vi "行列加减.vi"(10 "减":i32, 11 "加":dbl) -> (0 "x-3":i32, 1 "x-4":i32, 2 "x+4":dbl, 3 "x+3":dbl, 4 "x-2":i32, 5 "x+2":dbl, 6 "x-1":i32, 7 "x+1":dbl)   [LabVIEW 2018]
doc: "将行或列的索引位置进行加减以达到索引当前点周围点的目的。\n比如当前行列分别为5、5，为了查询它上一行同一列的点即4行5列的棋子，将其行减一变为4，列保持不变即为5。其它点同理对其进行索引。\n因要多次引用这个VI，因此加减的功能合在一个VI里面以供调用。"
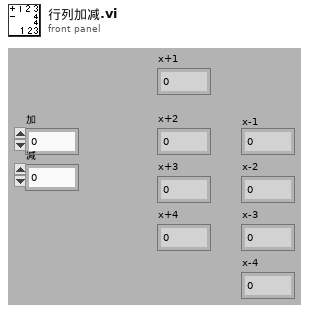
[diagram p1: front panel]
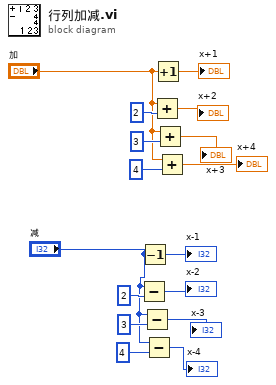
[diagram p0: block diagram]
diagram:
  n1 = Subtract(x="减", y=u8 2) -> (x-y=→"x-2":i32)
  n2 = Decrement(x="减") -> (x-1=→"x-1":i32)
  n3 = Subtract(x="减", y=u8 3) -> (x-y=→"x-3":i32)
  n4 = Subtract(x="减", y=u8 4) -> (x-y=→"x-4":i32)
  n5 = Add(x="加", y=u8 2) -> (x+y=→"x+2":dbl)
  n6 = Increment(x="加") -> (x+1=→"x+1":dbl)
  n7 = Add(x="加", y=u8 3) -> (x+y=→"x+3":dbl)
  n8 = Add(x="加", y=u8 4) -> (x+y=→"x+4":dbl)
